vi "Grab.vi"(8 "error in (no error)":errorcluster, 10 "Grab Toggle?":bool, 11 "Hatch Concrete in":refnum<class "Hatch Concrete.lvclass">) -> (0 "error out":errorcluster, 2 "Solenoid On?":bool, 3 "Hatch Concrete out":refnum<class "Hatch Concrete.lvclass">)   [LabVIEW 2019, in "Hatch.lvlib" / "Hatch Concrete.lvclass"]
doc: "This VI , stores the state of the hatch. The VI also commands whether the birdbeak should be open or close."
uses:
  Hatch Concrete.lvclass
  Hatch Concrete.lvclass/Hatch Concrete.ctl
  <vilib>/Rock Robotics/Network Tables/NT Write Boolean.vi
  Hatch.lvclass
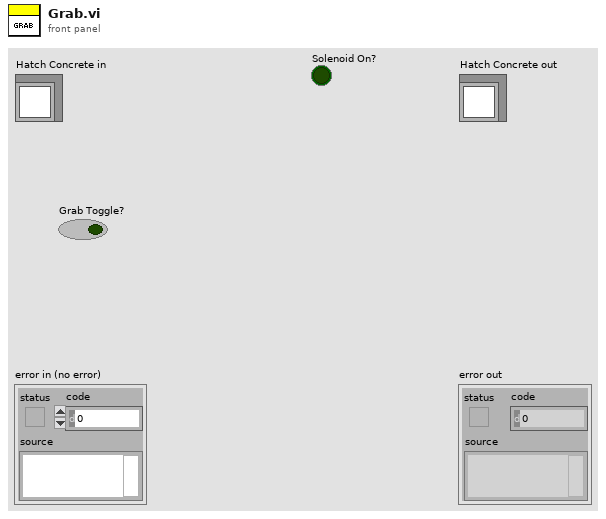
[diagram p1: front panel]
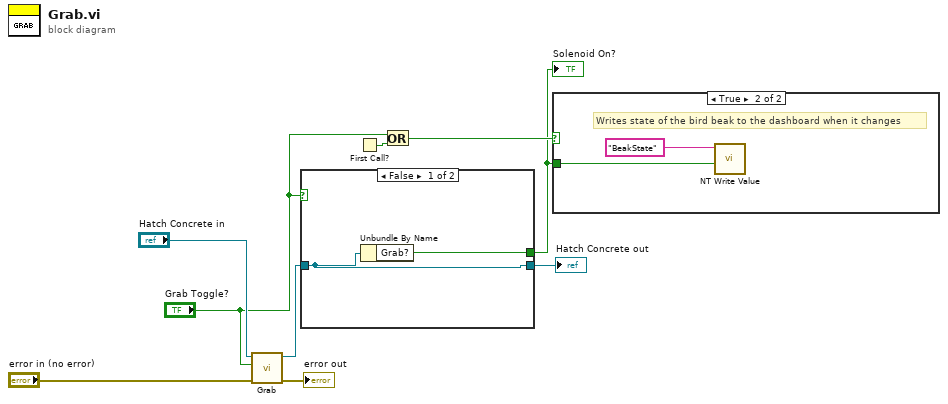
[diagram p0: block diagram]
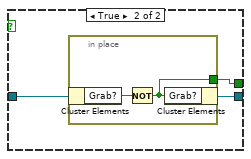
[diagram p3: hidden frame]
diagram:
  n1 = call-parent "Grab.vi"("error in (no error)"="error in (no error)", "Grab Toggle?"="Grab Toggle?", "Hatch in"="Hatch Concrete in") -> ("error out"=→"error out":errorcluster, "Hatch out"=w6:refnum<class "Hatch Concrete.lvclass">)  [unwired: 6 in, 1 out]
  n2 = case shown="False" "Grab Toggle?" {
    tunnel: [w10 w14] -> w5
    tunnel: [w11 w13] -> w1
    tunnel: w6 -> [w10 w12]
    frame False {
      n3 = Unbundle By Name(w10) -> ("Grab?"=w11:bool)
    }
    frame True {
      n4 = in-place {
        in-place-border: [w15] -> w13
        n5 = in-place-cluster #1(w12) -> ("Grab?"=w16:bool)
        n6 = Not(x=w16) -> (.not. x?=w15:bool)
        n7 = in-place-cluster #1("Grab?"=w15) -> (w14:refnum<class "Hatch Concrete.lvclass">)
      }
    }
  }
  "Hatch Concrete out" <- w5
  "Solenoid On?" <- w1
  n8 = First Call?() -> (First Call?: T/F=w3:bool)
  n9 = Or(x="Grab Toggle?", y=w3) -> (x .or. y?=w4:bool)
  n10 = case shown="True" w4 {
    tunnel: w1 -> [_ w18]
    frame False {
    }
    frame True {
      # "Writes state of the bird beak to the dashboard when it changes"
      n11 = call-poly <vilib>:"NT Write Value.vi"("Boolean"=w18, "Name"="BeakState") -> ()  [unwired: 9 in, 1 out]
    }
  }
